vi "Read Сontinuously Measured Values.vi"(8 "error in (no error)":errorcluster, 11 "VGC in":refnum<class "PL Inficon VGC.lvclass">) -> (0 "error out":errorcluster, 2 "measured values":cluster{"status":u16, "value":dbl}[][](array[cluster]) {"status" items=["data ok", "underrange", "overrange", "sensor error", "sensor off", "no sensor", "identification error", "error BPG, HPG, BCG"]; "value" format="%#_4p"}, 3 "VGC out":refnum<class "PL Inficon VGC.lvclass">)   [LabVIEW 2015, in "PL Inficon VGC.lvclass"]
doc: "Reads continuously measured values. Continuous output should be started prior to calling this VI."
uses:
  PL Inficon VGC.lvclass
  PL Inficon VGC.lvclass/PL Inficon VGC.ctl
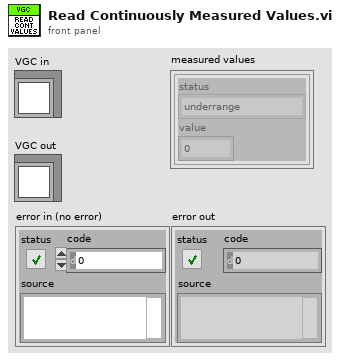
[diagram p1: front panel]
types:
  T1 = enum16{"Standard", "Buffered", "CRLF", "Immediate"}
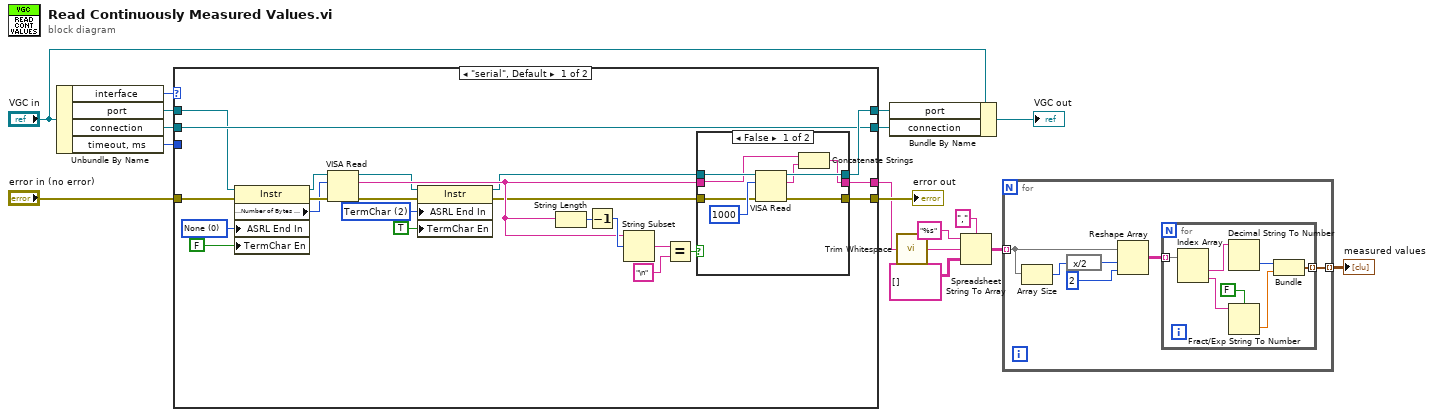
[diagram p0: block diagram]
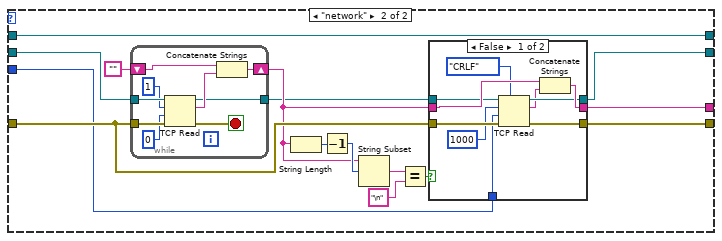
[diagram p3: hidden frame]
diagram:
  n1 = Unbundle By Name("VGC in") -> ("interface"=w12:enum16{"serial", "network"}, "port"=w17:refnum<visa-resource-name>, "connection"=w16:refnum<k5>, "timeout, ms"=w15:u32)
  n2 = case shown="\"serial\", Default" w12 {
    tunnel: [w40 w58] -> w3
    tunnel: w17 -> [w36 w66]
    tunnel: w16 -> [w37 w65]
    tunnel: [w39 w66] -> w14
    tunnel: w15 -> [_ w53]
    tunnel: [w37 w52] -> w13
    tunnel: [w38 w59] -> w2
    tunnel: "error in (no error)" -> [w35 w57]
    frame "serial", Default {
      w20 = u16 2 items=["None", "Last Bit", "TermChar"] ("Serial Settings:End Mode for Reads")
      w21 = u16 0 items=["None", "Last Bit", "TermChar"] ("Serial Settings:End Mode for Reads")
      n3 = property class="Instr"(reference=w36, error in=w35, "ASRL End In"=w21, "TermChar En"=FALSE ("Message Based Settings:Termination Character Enable")) -> (reference out=w22:refnum<visa-resource-name>, error out=w34:errorcluster, "Serial Settings:Number of Bytes at Serial Port"=w33:u32)
      n4 = VISA Read(VISA resource name=w22, byte count=w33, error in (no error)=w34) -> (VISA resource name out=w25:refnum<visa-resource-name>, read buffer=w27:string, error out=w26:errorcluster)  [unwired: 1 out]
      n5 = property class="Instr"(reference=w25, error in=w26, "ASRL End In"=w20, "TermChar En"=TRUE ("Message Based Settings:Termination Character Enable")) -> (reference out=w24:refnum<visa-resource-name>, error out=w23:errorcluster)
      n6 = String Length(string=w27) -> (length=w32:i32)
      n7 = Decrement(x=w32) -> (x-1=w31:i32)
      n8 = String Subset(string=w27, offset (0)=w31) -> (substring=w30:string)  [unwired: 1 in]
      n9 = Equal?(x=w30, y="\n") -> (x = y?=w28:bool)
      n10 = case shown="False" w28 {
        tunnel: [w47 w49] -> w40
        tunnel: [w46 w51] -> w39
        tunnel: [w41 w50] -> w38
        tunnel: w23 -> [w45 w49]
        tunnel: w24 -> [w44 w51]
        tunnel: w27 -> [w42 w50]
        frame False {
          n11 = VISA Read(VISA resource name=w44, byte count=u32 1000, error in (no error)=w45) -> (VISA resource name out=w46:refnum<visa-resource-name>, read buffer=w43:string, error out=w47:errorcluster)  [unwired: 1 out]
          n12 = Concatenate Strings(w42, w43) -> (w41:string)
        }
        frame True {
        }
      }
    }
    frame "network" {
      n13 = while {
        tunnel: w57 -> [w88]
        tunnel: w65 -> [w87]
        tunnel: [w83] -> w54
        shift-right: [w84] -> w55
        shift-left: "" -> [w80]
        stop <- w86 stop-if-true
        n14 = TCP Read(connection ID=w87, bytes to read=1, error in (no error)=w88, 9:0 ("timeout ms (25000)")) -> (connection ID out=w83:refnum<k5>, data out=w85:string, error out=w86:errorcluster)  [unwired: 1 in]
        n15 = Concatenate Strings(w80, w85) -> (w84:string)
      }
      n16 = String Length(string=w55) -> (length=w63:i32)
      n17 = Decrement(x=w63) -> (x-1=w62:i32)
      n18 = String Subset(string=w55, offset (0)=w62) -> (substring=w61:string)  [unwired: 1 in]
      n19 = Equal?(x=w61, y="\n") -> (x = y?=w56:bool)
      n20 = case shown="False" w56 {
        tunnel: [w73 w77] -> w58
        tunnel: [w74 w79] -> w52
        tunnel: [w75 w78] -> w59
        tunnel: w57 -> [w72 w77]
        tunnel: w54 -> [w70 w79]
        tunnel: w55 -> [w76 w78]
        tunnel: w53 -> [w69 _]
        frame False {
          n21 = TCP Read(connection ID=w70, bytes to read=1000 ("byte count"), error in (no error)=w72, 7:T1."CRLF" ("mode (standard)"), 9:w69) -> (connection ID out=w74:refnum<k5>, data out=w68:string, error out=w73:errorcluster)
          n22 = Concatenate Strings(w76, w68) -> (w75:string)
        }
        frame True {
        }
      }
    }
  }
  "error out" <- w3
  n23 = Bundle By Name(cluster="VGC in", "port"=w14, "connection"=w13) -> (→"VGC out":refnum<class "PL Inficon VGC.lvclass">)
  n24 = call <vilib>:"Trim Whitespace.vi"("string"=w2) -> ("trimmed string"=w1:string)  [unwired: 1 in]
  n25 = Spreadsheet String To Array(delimiter (Tab)=",", format string="%s", spreadsheet string=w1, array type (2D Dbl)=string[][] []) -> (array=w11:string[][])
  n26 = for {
    tunnel: w11 -> [w94] mode=indexing
    tunnel: [w89] -> w7 mode=indexing
    n27 = Array Size(array=w94) -> (size(s)=w93:i32)
    n28 = expression code="x/2"(w93) -> (w92:i32)
    n29 = Reshape Array(w94, w92, 2 ("dimension size")) -> (w90:string[][])
    n30 = for {
      tunnel: w90 -> [w101] mode=indexing
      tunnel: [w95] -> w89 mode=indexing
      n31 = Index Array(array=w101) -> (element #1=w98:string, element #2=w99:string)  [unwired: 2 in]
      n32 = Decimal String To Number(string=w98) -> (number=w97:i32)  [unwired: 2 in, 1 out]
      n33 = Fract/Exp String To Number(use system decimal point (T)=FALSE, string=w99) -> (number=w96:dbl)  [unwired: 2 in, 1 out]
      n34 = Bundle(w97, w96) -> (w95:cluster{i32, dbl})  [unwired: 1 in]
    }
  }
  "measured values" <- w7
